vi "UHR-Fleezers Control (host) - 11.9c.vi"() -> ()   [LabVIEW 2014] (continued)
                  }
                  frame True {
                    n2358 = flat-sequence {
                      tunnel: w3436 -> [w3439]
                      tunnel: [w3437] -> w3435
                      tunnel: w3435 -> [w3441]
                      frame #0 {
                        w3438 = TRUE ("Resize to Image Size? (Y)")
                        w3437 = 0 ("Window Number (0...15)")
                        n2359 = call "IMAQ WindNonTearing"("Window Number"=w3437, "NonTearing? (True)"=w3438) -> ()  [unwired: 8 in, 2 out]
                        n2360 = call "IMAQ WindDraw"("Resize to Image Size? (Y)"=w3438, "Window Number (0...15)"=w3437, "Image"=w3439) -> ()  [unwired: 7 in, 2 out]
                      }
                      frame #1 {
                        n2361 = call "IMAQ WindSize"("Scrollbars? (N)"=FALSE, "Width & Height"="Initial Window Size", "Window Number"=w3441) -> ()  [unwired: 3 in, 3 out]
                        n2362 = call "IMAQ WindMove"("Window Number (0...15)"=w3441, "Coordinates (screen)"="Initial Window Position") -> ()  [unwired: 3 in, 2 out]
                      }
                    }
                  }
                }
              }
              frame Enabled {
              }
            }
            n2363 = To Unsigned Byte Integer(number=w3386) -> (unsigned 8bit integer=w3385:u8[][])
            n2364 = call "IMAQ ArrayToImage"("Image Pixels (U8)"=w3385, "Image"=w3382) -> ("Image Out"=w3380:T2)  [unwired: 4 in, 5 out]
            n2365 = case shown="True" "Save Video" {
              tunnel: w3387 -> [_ w3445]
              tunnel: w3380 -> [_ w3444]
              frame False {
              }
              frame True {
                n2366 = call "IMAQ AVI Write Frame"("Image"=w3444, "Avi Refnum"=w3445) -> ()  [unwired: 2 in, 8 out]
              }
            }
            n2367 = case shown="True" "Save Image" {
              tunnel: w3385 -> [_ w3460]
              tunnel: w3384 -> [_ w3459]
              frame False {
              }
              frame True {
                n2368 = call <vilib>:"Flatten Pixmap.vi"("colors"=w3459, "8-bit pixmap"=w3460) -> ("image data"=w3466:T35)  [unwired: 4 in, 5 out]
                n2369 = call "Create new save file.vi"("Insert"="video_frame_" ("string"), "Ext"=".bmp" ("string"), "Index In"="Image Index") -> ("Path Out"=w3462:path, "Index Out"=w3467:dbl)
                n2370 = Increment(x=w3467) -> (x+1=w3461:dbl)
                n2371 = local write "Image Index"(w3461) -> ()
                n2372 = call <vilib>:"Write BMP File.vi"("image data"=w3466, "path to BMP file"=w3462) -> ()  [unwired: 1 in, 9 out]
              }
            }
            n2373 = case shown="True" "Target" {
              tunnel: w3380 -> [w3406 w3410]
              tunnel: [w3406 w3408] -> w3379
              frame False {
              }
              frame True {
                n2374 = local read "Target coordinates"() -> (w3407:cluster{"X1":dbl, "Y1":dbl, "X2":dbl, "Y2":dbl})
                n2375 = call "IMAQ Overlay Oval"("Color"=u32 16711680, "Bounding Rectangle"=w3407, "Image"=w3410) -> ("Image Out"=w3408:T2)  [unwired: 7 in, 1 out]
              }
            }
            "Primary Video Display" <- w3379
          }
        }
        n2376 = node-c288(w3341) -> ()  [unwired: 1 out]
      }
      n2377 = node-c288(w3325) -> ()  [unwired: 1 out]
      n2378 = call "DMR_CloseDevice2.vi"("driver handle IN"=w3330) -> ()  [unwired: 1 in, 4 out]
    }
    frame #4 {
      n2379 = call "DMR_Close.vi"() -> ()  [unwired: 1 out]
    }
  }
  n2380 = local write "Offset (nm)"(0.0 ("Offset (nm)")) -> ()
  n2381 = local write "Bead Mean (nm)"(0.0 ("Bead Mean (nm)")) -> ()
  n2382 = local write "Total Volume\nFlowed P1 (uL)"(w26) -> ()
  n2383 = local write "Total Volume\nFlowed Samp (uL)"(w26) -> ()
  n2384 = local write "Total Volume\nFlowed P3 (uL)"(w26) -> ()
  n2385 = node-c288(i64 1 ("Period"), 1 ("Processor")) -> (w200:T22)  [unwired: 2 out]
  n2386 = timed-loop "Acquire Data" {
    tunnel: w32 -> [w3775]
    tunnel: w79 -> [w3774]
    tunnel: [w3804] -> w293
    tunnel: [w3799] -> w291
    timing: w200 -> [_]
    timing-out: [_] -> w199
    tunnel: w98 -> [w3614]
    stop <- "Stop All" stop-if-true
    w3532 = "Initialize"
    w3601 = "NI_ChannelName" ("name")
    # "I think that the conversion\nfrom 'wiggle amp' to nm\nis 0.277 nm/input. So, 1000\nfor an input is 277 nm."
    n2387 = node-c288() -> ()  [unwired: 2 out]
    n2388 = First Call?() -> (First Call?: T/F=w3567:bool)
    n2389 = Or(x="Reset", y=w3567) -> (x .or. y?=w3568:bool)
    n2390 = local read "Flushing P1"() -> (w3487:bool)
    n2391 = case "Reset data stream" shown="True" w3568 {
      tunnel: w3775 -> [w4844 w4852]
      tunnel: w3774 -> [w4843 w4851]
      tunnel: [w4844 w4846] -> w3480
      tunnel: [w4843 w4845] -> w3770
      frame False {
      }
      frame True {
        w4849 = TRUE ("AI to FIFO")
        n2392 = local write "Overflow (data lost)"(FALSE ("Overflow (data lost)")) -> ()
        n2393 = call "reset FPGA DMA.vi"("error in"=w4851, "FPGA VI Reference In"=w4852) -> ("error out"=w4847:errorcluster, "FPGA VI Reference Out"=w4848:T20)
        n2394 = xnode "Read/Write Control"("FPGA VI Reference In"=w4848, "error in"=w4847, "AI to FIFO"=w4849, "APD to FIFO"=w4849) -> ("FPGA VI Reference Out"=w4846:T20, "error out"=w4845:errorcluster)
      }
    }
    n2395 = case shown="True" w3487 {
      frame False {
      }
      frame True {
        n2396 = local read "Flush rate (uL/m) P1"() -> (w3877:dbl)
        n2397 = local read "HP1 Flush Time (s)"() -> (w3883:dbl)
        n2398 = local read "DMA Update Period (s)"() -> (w3870:dbl)
        n2399 = Divide(x=w3877, y=60.0) -> (x/y=w3869:dbl)
        n2400 = feedback #4(0.0) -> (w3872:dbl)
        n2401 = Divide(x=w3883, y=w3870) -> (x/y=w3875:dbl)
        n2402 = feedback #5(0) -> (w3881:i32)
        n2403 = Increment(x=w3881) -> (x+1=w3874:i32)
        n2404 = Multiply(x=w3870, y=w3869) -> (x*y=w3868:dbl)
        n2405 = Greater?(x=w3874, y=w3875) -> (0:w3880:bool)
        n2406 = Compound Arithmetic op=MULTIPLY(w3870, w3874, w3869) -> (→"P1 Flush Volume (uL)":dbl)
        n2407 = Divide(x=w3874, y=w3875) -> (x/y=→"P1 Flushing Bar":dbl)
        n2408 = Add(x=w3868, y=w3872) -> (x+y=w3871:dbl)
        "Total Volume\nFlowed P1 (uL)" <- w3871
        n2409 = feedback-in #4(w3871) -> ()
        n2410 = case shown="True" w3880 {
          tunnel: w3874 -> [w3884 _]
          tunnel: [w3884 0] -> w3879
          frame False {
          }
          frame True {
            w3885 = FALSE ("Flushing P1")
            n2411 = local write "Inject Pump 1"(w3885) -> ()
            n2412 = local write "Flushing P1"(w3885) -> ()
            n2413 = property on="Clear Volume P1" class="Bool (strict)"("Val(Sgnl)"=TRUE ("Value (Signaling)")) -> ()  [unwired: 2 in, 2 out]
          }
        }
        n2414 = feedback-in #5(w3879) -> ()
      }
    }
    n2415 = Or(x="Start AOD Scan", y="Trap Raster Scan") -> (x .or. y?=w3722:bool)
    n2416 = case "Start AOM raster scan" shown="True" w3722 {
      tunnel: w3480 -> [w4694 w4704]
      tunnel: w3770 -> [w4693 w4703]
      tunnel: [w4694 w4697] -> w3472
      tunnel: [w4693 w4696] -> w3769
      frame False {
      }
      frame True {
        n2417 = case shown="True" "Restart DMA? (AOD)" {
          tunnel: [w4742 w4744] -> w4698
          tunnel: [w4741 w4743] -> w4699
          tunnel: w4704 -> [w4742 w4746]
          tunnel: w4703 -> [w4741 w4745]
          frame False {
          }
          frame True {
            n2418 = local write "Overflow (data lost)"(FALSE ("Overflow (data lost)")) -> ()
            n2419 = call "reset FPGA DMA.vi"("error in"=w4745, "FPGA VI Reference In"=w4746) -> ("error out"=w4743:errorcluster, "FPGA VI Reference Out"=w4744:T20)
          }
        }
        n2420 = local write "Trap Raster Scan"(FALSE ("Trap Raster Scan")) -> ()
        n2421 = case shown="False" "Move MCL Also?" {
          tunnel: w4699 -> [w4708 w4736]
          tunnel: w4698 -> [w4709 w4737]
          tunnel: [w4707 w4740] -> w4697
          tunnel: [w4706 w4739] -> w4696
          frame False {
            w4705 = TRUE ("AI to FIFO")
            n2422 = xnode "Read/Write Control"("FPGA VI Reference In"=w4709, "error in"=w4708, "AI to FIFO"=w4705, "APD to FIFO"=w4705, "Start scan"=w4705) -> ("FPGA VI Reference Out"=w4707:T20, "error out"=w4706:errorcluster)
          }
          frame True {
            w4733 = FALSE ("1D or 2D Scan?")
            w4738 = TRUE ("AI to FIFO")
            # "Count for MCL loop"
            # "N total cycles"
            # "N steps"
            # "V_int"
            n2423 = local read "Scan Range (nm)"() -> (w4715:dbl)
            n2424 = local read "Number of F/B Scans (AOD)"() -> (w4732:u16)
            n2425 = Sign(1:w4715) -> (0:w4714:dbl)
            n2426 = Compound Arithmetic op=MULTIPLY(w4715, "MCL Step Position Ratio", "MCL/AOM Scale Tweak") -> (w4719:dbl)
            n2427 = Negate(x=w4714) -> (-x=w4711:dbl)
            n2428 = Multiply(x=w4711, y="MCL Step Increment (V_int)") -> (x*y=w4713:dbl)
            n2429 = Divide(x=w4719, y="MCL X Cal (nm/V)") -> (x/y=w4725:dbl)
            n2430 = Multiply(x=32767.0 ("y"), y=w4725) -> (x*y=w4731:dbl)
            n2431 = local read "Total Counts (ticks)"() -> (w4716:u32)
            n2432 = local read "Cycles/step (AOD)"() -> (w4727:u64)
            n2433 = local read "Scan steps (AOD)"() -> (w4728:u64)
            n2434 = Divide(x=w4731, y=10.0) -> (x/y=w4724:dbl)
            n2435 = Divide(x=w4724, y="MCL Step Increment (V_int)") -> (x/y=w4722:dbl)
            n2436 = Absolute Value(x=w4722) -> (abs(x)=w4710:dbl)
            n2437 = Compound Arithmetic op=MULTIPLY(w4728, w4727, w4716) -> (w4723:u64)
            n2438 = local write "wait to reset values"(w4738) -> ()
            n2439 = local write "MCL Scanning"(w4738) -> ()
            n2440 = Divide(x=w4723, y=w4710) -> (x/y=w4720:dbl)
            "MCL Count" <- w4720
            n2441 = xnode "Read/Write Control"("FPGA VI Reference In"=w4737, "error in"=w4736, "Scan steps (MCL)"=w4710, "Number of scans (MCL)"=w4732, "Cycles per step (MCL)"=u64 1, "Scan freq.  increment (MCL)"=w4713, "1D or 2D Scan?"=w4733, "MCL Scan Axis"=w4733, "Cont. Scan (MCL)"=w4733, "MCL count"=w4720) -> ("FPGA VI Reference Out"=w4735:T20, "error out"=w4734:errorcluster)
            n2442 = xnode "Read/Write Control"("FPGA VI Reference In"=w4735, "error in"=w4734, "AI to FIFO"=w4738, "APD to FIFO"=w4738, "Start scan"=w4738, "Start scan (MCL)"=w4738) -> ("FPGA VI Reference Out"=w4740:T20, "error out"=w4739:errorcluster)
          }
        }
        "Raster Scanning..." <- TRUE ("Scanning...")
      }
    }
    n2443 = local read "Flushing P3"() -> (w3488:bool)
    n2444 = case "Keep track of when Harvard Pump 3 is done flushing" shown="True" w3488 {
      frame False {
      }
      frame True {
        n2445 = local read "Flush rate (uL/m) P3"() -> (w3896:dbl)
        n2446 = local read "DMA Update Period (s)"() -> (w3890:dbl)
        n2447 = local read "HP3 Flush Time (s)"() -> (w3904:dbl)
        n2448 = Divide(x=w3896, y=60.0) -> (x/y=w3891:dbl)
        n2449 = feedback #6(0) -> (w3902:i32)
        n2450 = Increment(x=w3902) -> (x+1=w3897:i32)
        n2451 = Divide(x=w3904, y=w3890) -> (x/y=w3898:dbl)
        n2452 = Multiply(x=w3890, y=w3891) -> (x*y=w3889:dbl)
        n2453 = Greater?(x=w3897, y=w3898) -> (0:w3901:bool)
        n2454 = feedback #7(0.0) -> (w3892:dbl)
        n2455 = Compound Arithmetic op=MULTIPLY(w3890, w3897, w3891) -> (→"P3 Flush Volume (uL)":dbl)
        n2456 = case shown="True" w3901 {
          tunnel: w3897 -> [w3905 _]
          tunnel: [w3905 0] -> w3900
          frame False {
          }
          frame True {
            w3906 = FALSE ("Flushing P3")
            n2457 = local write "Inject Pump 3"(w3906) -> ()
            n2458 = local write "Flushing P3"(w3906) -> ()
            n2459 = property on="Clear Volume P3" class="Bool (strict)"("Val(Sgnl)"=TRUE ("Value (Signaling)")) -> ()  [unwired: 2 in, 2 out]
          }
        }
        n2460 = feedback-in #6(w3900) -> ()
        n2461 = Divide(x=w3897, y=w3898) -> (x/y=→"P3 Flushing Bar":dbl)
        n2462 = Add(x=w3889, y=w3892) -> (x+y=w3893:dbl)
        "Total Volume\nFlowed P3 (uL)" <- w3893
        n2463 = feedback-in #7(w3893) -> ()
      }
    }
    n2464 = And(x="Save scans", y=w3722) -> (x .and. y?=w3768:bool)
    n2465 = local read "Flushing samp"() -> (w3481:bool)
    n2466 = case shown="True" w3481 {
      frame False {
      }
      frame True {
        n2467 = local read "DMA Update Period (s)"() -> (w3849:dbl)
        n2468 = local read "Flush rate (mL/m)"() -> (w3861:dbl)
        n2469 = local read "Samp Flush Time (s)"() -> (w3862:dbl)
        n2470 = Divide(x=w3861, y=60.0) -> (x/y=w3848:dbl)
        n2471 = feedback #8(0) -> (w3854:i32)
        n2472 = Increment(x=w3854) -> (x+1=w3853:i32)
        n2473 = Divide(x=w3862, y=w3849) -> (x/y=w3858:dbl)
        n2474 = Multiply(x=w3849, y=w3848) -> (x*y=w3847:dbl)
        n2475 = Greater?(x=w3853, y=w3858) -> (0:w3857:bool)
        n2476 = feedback #9(0.0) -> (w3850:dbl)
        n2477 = Compound Arithmetic op=MULTIPLY(w3849, w3853, w3848) -> (→"Samp Volume (uL)":dbl)
        n2478 = Divide(x=w3853, y=w3858) -> (x/y=→"Samp flush bar":dbl)
        n2479 = case shown="True" w3857 {
          tunnel: [w3863 0] -> w3856
          tunnel: w3853 -> [w3863 _]
          frame False {
          }
          frame True {
            w3866 = FALSE ("Flushing samp")
            n2480 = local write "Sample Channel\nFlow"(w3866) -> ()
            n2481 = local write "Flushing samp"(w3866) -> ()
            n2482 = property on="Clear Volume" class="Bool (strict)"("Val(Sgnl)"=TRUE) -> ()  [unwired: 2 in, 2 out]
          }
        }
        n2483 = feedback-in #8(w3856) -> ()
        n2484 = Add(x=w3847, y=w3850) -> (x+y=w3851:dbl)
        "Total Volume\nFlowed Samp (uL)" <- w3851
        n2485 = feedback-in #9(w3851) -> ()
      }
    }
    n2486 = Compound Arithmetic op=OR("Start MCL Scan", "Confocal\nImage", "Confocal\nLinescan") -> (w3720:bool)
    n2487 = And(x="Save Data (MCL)", y=w3720) -> (x .and. y?=w3767:bool)
    n2488 = case "Start MCL raster scan" shown="True" w3720 {
      tunnel: w3472 -> [w4311 w4327]
      tunnel: w3769 -> [w4310 w4326]
      tunnel: [w4311 w4322] -> w3479
      tunnel: [w4310 w4321] -> w3477
      tunnel: [FALSE w4320] -> w3753
      tunnel: "Start MCL Scan" -> [_ w4315]
      tunnel: "Confocal\nImage" -> [_ w4314]
      tunnel: "Confocal\nLinescan" -> [_ _]
      frame False {
      }
      frame True {
        w4320 = TRUE
        n2489 = case shown="True" "Restart DMA? (MCL)" {
          tunnel: [w4372 w4374] -> w4325
          tunnel: [w4371 w4373] -> w4324
          tunnel: w4327 -> [w4372 w4377]
          tunnel: w4326 -> [w4371 w4376]
          frame False {
          }
          frame True {
            n2490 = call "reset FPGA DMA.vi"("error in"=w4376, "FPGA VI Reference In"=w4377) -> ("error out"=w4373:errorcluster, "FPGA VI Reference Out"=w4374:T20)
            n2491 = local write "Overflow (data lost)"(FALSE ("Overflow (data lost)")) -> ()
          }
        }
        n2492 = case shown="False" w4315 {
          selector: w4315 -> [_ w4331]
          tunnel: w4314 -> [w4330 _]
          tunnel: [w4330 w4331] -> w4313
          frame False {
            n2493 = property on="2D or 1D Scan" class="Bool (strict)"("Val(Sgnl)"=w4330) -> ()  [unwired: 2 in, 2 out]
            n2494 = property on="Confocal\nImage" class="Bool (strict)"("Value"=FALSE ("Start Confocal Map")) -> ()  [unwired: 2 in, 2 out]
          }
          frame True {
          }
        }
        n2495 = local write "MCL Scanning"(w4320) -> ()
        n2496 = local read "AO1"() -> (w4317:dbl)
        n2497 = local read "AO2"() -> (w4316:dbl)
        n2498 = case shown="True" "Center Scan" {
          tunnel: w4325 -> [w4338 w4370]
          tunnel: w4324 -> [w4337 w4369]
          tunnel: [w4336 w4368] -> w4322
          tunnel: [w4335 w4367] -> w4321
          tunnel: [w4333 w4354] -> w4319
          tunnel: [w4332 w4353] -> w4318
          tunnel: w4317 -> [w4333 w4359]
          tunnel: w4316 -> [w4332 w4362]
          tunnel: w4313 -> [_ _]
          frame False {
            w4334 = TRUE ("AI to FIFO")
            n2499 = xnode "Read/Write Control"("FPGA VI Reference In"=w4338, "error in"=w4337, "AI to FIFO"=w4334, "APD to FIFO"=w4334, "Start scan (MCL)"=w4334) -> ("FPGA VI Reference Out"=w4336:T20, "error out"=w4335:errorcluster)
          }
          frame True {
            w4366 = TRUE ("AI to FIFO")
            n2500 = local read "Scan steps (MCL)"() -> (w4345:u64)
            n2501 = local read "Scan lines (y)"() -> (w4341:u64)
            n2502 = local read "Fast Scan Dir"() -> (w4352:bool)
            n2503 = local read "Actual MCL Inc (V)"() -> (w4342:dbl)
            n2504 = Decrement(x=w4341) -> (x-1=w4340:u64)
            n2505 = Decrement(x=w4345) -> (x-1=w4344:u64)
            n2506 = Multiply(x=w4342, y=w4340) -> (x*y=w4339:dbl)
            n2507 = Divide(x=w4339, y=2.0) -> (x/y=w4349:dbl)
            n2508 = Multiply(x=w4342, y=w4344) -> (x*y=w4343:dbl)
            n2509 = Divide(x=w4343, y=2.0) -> (x/y=w4348:dbl)
            n2510 = Select(t=w4348, s=w4352, f=w4349) -> (s? t:f=w4347:dbl)
            n2511 = Select(t=w4349, s=w4352, f=w4348) -> (s? t:f=w4351:dbl)
            n2512 = Subtract(x=w4359, y=w4351) -> (x-y=w4350:dbl)
            n2513 = Subtract(x=w4362, y=w4347) -> (x-y=w4346:dbl)
            n2514 = local read "2D or 1D Scan"() -> (w4364:bool)
            n2515 = Not(x=w4352) -> (.not. x?=w4358:bool)
            n2516 = Not(x=w4364) -> (.not. x?=w4360:bool)
            n2517 = And(x=w4352, y=w4360) -> (x .and. y?=w4361:bool)
            n2518 = And(x=w4360, y=w4358) -> (x .and. y?=w4363:bool)
            n2519 = Select(t=w4362, s=w4363, f=w4346) -> (s? t:f=w4353:dbl)
            n2520 = Select(t=w4359, s=w4361, f=w4350) -> (s? t:f=w4354:dbl)
            n2521 = call "Volt to I16.vi"("Voltage In"=w4354) -> ("I16 Voltage Out"=w4357:i16)
            n2522 = call "Volt to I16.vi"("Voltage In"=w4353) -> ("I16 Voltage Out"=w4356:i16)
            n2523 = xnode "Read/Write Control"("FPGA VI Reference In"=w4370, "error in"=w4369, "AI to FIFO"=w4366, "APD to FIFO"=w4366, "Start scan (MCL)"=w4366, "AO1"=w4357, "AO2"=w4356) -> ("FPGA VI Reference Out"=w4368:T20, "error out"=w4367:errorcluster)
          }
        }
        "Initial Y" <- w4319
        "Initial X" <- w4318
        n2524 = local write "Tab Control 6"(T3."Imaging" ("Tab Control 6")) -> ()
        "wait to reset values" <- w4320
      }
    }
    n2525 = case shown="True" "Wiggle" {
      selector: "Wiggle" -> [w3820 _]
      tunnel: w3479 -> [w3822 w3835]
      tunnel: [w3819 w3838] -> w3478
      tunnel: w3477 -> [w3821 w3833]
      tunnel: [w3818 w3837] -> w3476
      frame False {
        n2526 = xnode "Read/Write Control"("FPGA VI Reference In"=w3822, "error in"=w3821, "Wiggle trap 1"=w3820) -> ("FPGA VI Reference Out"=w3819:T20, "error out"=w3818:errorcluster)
      }
      frame True {
        w3827 = FALSE ("Abort wiggle")
        w3831 = TRUE
        n2527 = local read "Restart DMA? (AOD)"() -> (w3836:bool)
        n2528 = case shown="True" w3836 {
          tunnel: w3835 -> [w3840 w3845]
          tunnel: [w3840 w3844] -> w3834
          tunnel: w3833 -> [w3839 w3843]
          tunnel: [w3839 w3842] -> w3832
          frame False {
          }
          frame True {
            n2529 = local write "Overflow (data lost)"(FALSE) -> ()
            n2530 = call "reset FPGA DMA.vi"("error in"=w3843, "FPGA VI Reference In"=w3845) -> ("error out"=w3842:errorcluster, "FPGA VI Reference Out"=w3844:T20)
          }
        }
        n2531 = local write "Wiggle"(FALSE) -> ()
        n2532 = xnode "Read/Write Control"("FPGA VI Reference In"=w3834, "error in"=w3832, "AI to FIFO"=w3831, "APD to FIFO"=w3831, "Wiggle trap 1"="Wiggle T1", "Wiggle freq 1 (Hz)"="Wiggle freq 1 (Hz)", "Wiggle amp 1"="Wiggle amp 1 (units?)", "Abort wiggle 1"=w3827, "Wiggle trap 2"="Wiggle T2", "Abort wiggle 2"=w3827, "Wiggle freq 2 (Hz)"="Wig Freq 2 (Hz)", "Wiggle amp 2"="Wig amp 2") -> ("FPGA VI Reference Out"=w3838:T20, "error out"=w3837:errorcluster)
      }
    }
    n2533 = local read "Trap Pos Elements/DMA read"() -> (w3610:u32)
    n2534 = local read "Trap AI Elements/DMA read"() -> (w3683:u32)
    n2535 = local read "APD Elements/DMA read"() -> (w3649:u32)
    n2536 = xnode "Get APD Data"("FPGA VI Reference In"=w3478, "error in"=w3476, "Number of Elements"=w3649, "Timeout (ms)"=-1) -> ("Data"=w3648:u32[], "Elements Remaining"=→"APD FIFO Elements Remaining":u32)  [unwired: 2 out]
    n2537 = xnode "Invoke Method"("FPGA VI Reference In"=w3478, "error in"=w3476, "Number of Elements"=w3610, "Timeout (ms)"=-1) -> ("Data"=w3574:u16[], "Elements Remaining"=→"Trap Pos FIFO El Remaining":u32)  [unwired: 2 out]
    n2538 = xnode "Get Trap Data"("FPGA VI Reference In"=w3478, "error in"=w3476, "Number of Elements"=w3683, "Timeout (ms)"=-1 ("Timeout")) -> ("FPGA VI Reference Out"=w3509:T20, "error out"=w3508:errorcluster, "Data"=w3575:i16[], "Elements Remaining"=w3812:u32)
    "FIFO El. Rem." <- w3812
    n2539 = local read "Trap AI FIFO Depth"() -> (w3814:u32)
    n2540 = Subtract(x=w3814, y=w3683) -> (x-y=w3813:u32)
    n2541 = Decimate 1D Array(w3574) -> (w3571:u16[], w3573:u16[], w3572:u16[])
    n2542 = Divide(x=w3812, y=w3813) -> (x/y=w3811:dbl)
    "Buffer Status" <- w3811
    n2543 = To Unsigned Long Integer(number=w3571) -> (unsigned 32bit integer=w3570:u32[])
    n2544 = Join Numbers(hi=w3573, lo=w3572) -> ((hi.lo)=w3569:u32[])
    n2545 = Equal?(x=w3811, y=1.0) -> (x = y?=w3809:bool)
    n2546 = Join Numbers(hi=w3570, lo=w3569) -> ((hi.lo)=w3563:u64[])
    n2547 = call "IR AOM word to freq - vec.vi"("Frequency Word In (double vec)"=w3563) -> ("Frequency Out"=w3609:dbl[])
    n2548 = case "Alert buffer overflow" shown="True" w3809 {
      frame False {
      }
      frame True {
        n2549 = call <vilib>:"Beep.vi"() -> ()  [unwired: 3 in, 9 out]
        "Overflow (data lost)" <- TRUE ("Overflow (data lost)")
      }
    }
    n2550 = Decimate 1D Array(w3609) -> (w3608:dbl[], w3607:dbl[])
    n2551 = Build Array(w3608, w3607) -> (w3606:dbl[][])
    n2552 = local read "Trap Sets"() -> (w3682:u32)
    n2553 = case "Deinterlace trap data, average down PSD" shown="2" w3682 {
      tunnel: w3575 -> [w4407 w4472]
      tunnel: [w4404 w4469] -> w3675
      tunnel: [w4407 w4471] -> w3566
      tunnel: "Detector Type" -> [w4406 w4467]
      tunnel: [w4405 w4470] -> w3674
      tunnel: [w4403 w4468] -> w3786
      frame 1, Default {
        n2554 = Divide(x=w4407, y=3276.7) -> (x/y=w4408:dbl[])
        n2555 = Decimate 1D Array(w4408) -> (w4417:dbl[], w4416:dbl[], w4415:dbl[], w4414:dbl[], w4413:dbl[], w4412:dbl[], w4411:dbl[], w4410:dbl[])
        n2556 = case shown="\"IR-QPD + PSD + FB-QPD position\"" w4406 {
          tunnel: w4417 -> [w4441 w4466]
          tunnel: w4416 -> [w4440 w4465]
          tunnel: w4415 -> [w4425 w4443]
          tunnel: w4414 -> [w4426 w4453]
          tunnel: w4413 -> [w4439 w4464]
          tunnel: w4412 -> [w4438 w4463]
          tunnel: w4411 -> [w4422 w4444]
          tunnel: w4410 -> [w4421 w4442]
          tunnel: [w4420 w4450] -> w4405
          tunnel: [w4419 w4449] -> w4404
          tunnel: [w4418 w4448] -> w4403
          frame "IR-QPD + PSD + FB-QPD", Default {
            w4418 = 0  # Channel pattern
            n2557 = Divide(x=w4441, y=w4426) -> (x/y=w4428:dbl[])
            n2558 = Divide(x=w4440, y=w4426) -> (x/y=w4427:dbl[])
            n2559 = Divide(x=w4439, y=w4422) -> (x/y=w4424:dbl[])
            n2560 = Divide(x=w4438, y=w4421) -> (x/y=w4423:dbl[])
            n2561 = Build Array(w4428, w4427, w4426, w4425, w4424, w4423, w4422, w4421) -> (w4419:dbl[][])
            n2562 = Bundle("T1 Y", "T1 X", "T1 Sum", "FB Sum", "PSD Y", "PSD X", "PSD Y Sum", "PSD X Sum") -> (w4437:T42)  [unwired: 1 out]
            n2563 = Cluster To Array(cluster=w4437) -> (array=w4420:string[])
          }
          frame "IR-QPD + PSD + FB-QPD position" {
            w4448 = 3  # Channel pattern
            n2564 = Negate(x=w4444) -> (-x=w4445:dbl[])
            n2565 = Divide(x=w4466, y=w4453) -> (x/y=w4455:dbl[])
            n2566 = Divide(x=w4465, y=w4453) -> (x/y=w4454:dbl[])
            n2567 = Divide(x=w4464, y=w4444) -> (x/y=w4452:dbl[])
            n2568 = Divide(x=w4463, y=w4445) -> (x/y=w4451:dbl[])
            n2569 = Build Array(w4455, w4454, w4453, w4442, w4443, w4452, w4451, w4444) -> (w4449:dbl[][])
            n2570 = Bundle("T1 Y", "T1 X", "T1 Sum", "FB X", "FB Sum", "PSD Y", "PSD X", "PSD Y Sum") -> (w4462:T42)  [unwired: 1 out]
            n2571 = Cluster To Array(cluster=w4462) -> (array=w4450:string[])
          }
        }
      }
      frame 2 {
        n2572 = case shown="\"IR-QPD + PSD + FB-QPD\", Default" w4467 {
          tunnel: w4472 -> [w4534 w4601 w4672]
          tunnel: [w4473 w4592 w4603] -> w4471
          tunnel: [w4500 w4583 w4650] -> w4470
          tunnel: [w4499 w4546 w4617] -> w4469
          tunnel: [w4493 w4581 w4648] -> w4468
          frame "IR-QPD + PSD + FB-QPD", Default {
            w4493 = 1  # Channel pattern
            # "time average x2 the 4th signal and the 4 psd signals (detection laser)"
            # "deinterlace 3 signals from qpd"
            n2573 = Decimate 1D Array(w4534) -> (w4533:i16[], w4532:i16[], w4498:i16[], w4531:i16[], w4521:i16[], w4519:i16[], w4518:i16[], w4516:i16[])
            n2574 = Decimate 1D Array(w4498) -> (w4497:i16[], w4496:i16[])
            n2575 = Decimate 1D Array(w4533) -> (w4530:i16[], w4502:i16[])
            n2576 = Decimate 1D Array(w4532) -> (w4529:i16[], w4527:i16[])
            n2577 = Decimate 1D Array(w4531) -> (w4528:i16[], w4526:i16[])
            n2578 = call "downsample 1D array - double.vi"("Ave N"=2.0, "Array In"=w4521) -> ("Array Out"=w4520:dbl[])  [unwired: 1 out]
            n2579 = call "downsample 1D array - double.vi"("Ave N"=2.0, "Array In"=w4519) -> ("Array Out"=w4501:dbl[])  [unwired: 1 out]
            n2580 = call "downsample 1D array - double.vi"("Ave N"=2.0, "Array In"=w4518) -> ("Array Out"=w4517:dbl[])  [unwired: 1 out]
            n2581 = call "downsample 1D array - double.vi"("Ave N"=2.0, "Array In"=w4516) -> ("Array Out"=w4515:dbl[])  [unwired: 1 out]
            n2582 = Interleave 1D Arrays(w4530, w4529, w4528, w4502, w4527, w4526, w4497, w4496, w4520, w4501, w4517, w4515) -> (w4514:dbl[])
            n2583 = Divide(x=w4514, y=3276.7) -> (x/y=w4513:dbl[])
            n2584 = Decimate 1D Array(w4513) -> (w4512:dbl[], w4511:dbl[], w4510:dbl[], w4509:dbl[], w4508:dbl[], w4507:dbl[], w4495:dbl[], w4494:dbl[], w4506:dbl[], w4505:dbl[], w4504:dbl[], w4503:dbl[])
            n2585 = Divide(x=w4512, y=w4510) -> (x/y=w4480:dbl[])
            n2586 = Divide(x=w4511, y=w4510) -> (x/y=w4479:dbl[])
            n2587 = Divide(x=w4509, y=w4507) -> (x/y=w4478:dbl[])
            n2588 = Divide(x=w4508, y=w4507) -> (x/y=w4477:dbl[])
            n2589 = Divide(x=w4506, y=w4504) -> (x/y=w4476:dbl[])
            n2590 = Divide(x=w4505, y=w4503) -> (x/y=w4475:dbl[])
            n2591 = Build Array(w4480, w4479, w4510, w4478, w4477, w4507, w4495, w4494, w4476, w4475, w4504, w4503) -> (w4499:dbl[][])
            n2592 = Bundle("T1 Y", "T1 X", "T1 Sum", "T2 Y", "T2 X", "T2 Sum", "T1 FB Sum", "T2 FB Sum", "PSD Y", "PSD X", "PSD Y Sum", "PSD X Sum") -> (w4481:T43)  [unwired: 1 out]
            n2593 = To Word Integer(number=w4514) -> (16bit integer=w4473:i16[])
            n2594 = Cluster To Array(cluster=w4481) -> (array=w4500:string[])
          }
          frame "IR-QPD + PSD + FB-QPD X position" {
            w4581 = 2  # Channel pattern
            # "time average x2 the 3 psd signals (detection laser)"
            # "deinterlace 3 signals from qpds"
            n2595 = Decimate 1D Array(w4601) -> (w4600:i16[], w4599:i16[], w4582:i16[], w4598:i16[], w4544:i16[], w4541:i16[], w4538:i16[], w4569:i16[])
            n2596 = Decimate 1D Array(w4582) -> (w4567:i16[], w4565:i16[])
            n2597 = Decimate 1D Array(w4600) -> (w4597:i16[], w4584:i16[])
            n2598 = Decimate 1D Array(w4599) -> (w4596:i16[], w4594:i16[])
            n2599 = Decimate 1D Array(w4598) -> (w4595:i16[], w4593:i16[])
            n2600 = Decimate 1D Array(w4569) -> (w4568:i16[], w4566:i16[])
            n2601 = call "downsample 1D array - I16.vi"("Ave N"=2.0, "Array In"=w4544) -> ("Array Out"=w4542:i16[])  [unwired: 1 in]
            n2602 = call "downsample 1D array - I16.vi"("Ave N"=2.0, "Array In"=w4538) -> ("Array Out"=w4536:i16[])  [unwired: 1 in]
            n2603 = call "downsample 1D array - I16.vi"("Ave N"=2.0, "Array In"=w4541) -> ("Array Out"=w4539:i16[])  [unwired: 1 in]
            n2604 = Interleave 1D Arrays(w4597, w4596, w4595, w4584, w4594, w4593, w4568, w4567, w4566, w4565, w4542, w4539, w4536) -> (w4592:i16[])
            n2605 = Divide(x=w4592, y=3276.7) -> (x/y=w4591:dbl[])
            n2606 = Decimate 1D Array(w4591) -> (w4590:dbl[], w4589:dbl[], w4588:dbl[], w4587:dbl[], w4586:dbl[], w4585:dbl[], w4557:dbl[], w4555:dbl[], w4554:dbl[], w4552:dbl[], w4551:dbl[], w4550:dbl[], w4547:dbl[])
            n2607 = Negate(x=w4547) -> (-x=w4545:dbl[])
            n2608 = Divide(x=w4551, y=w4547) -> (x/y=w4549:dbl[])
            n2609 = Divide(x=w4550, y=w4545) -> (x/y=w4548:dbl[])
            n2610 = Divide(x=w4590, y=w4588) -> (x/y=w4573:dbl[])
            n2611 = Divide(x=w4589, y=w4588) -> (x/y=w4572:dbl[])
            n2612 = Divide(x=w4587, y=w4585) -> (x/y=w4571:dbl[])
            n2613 = Divide(x=w4586, y=w4585) -> (x/y=w4570:dbl[])
            n2614 = Divide(x=w4557, y=w4555) -> (x/y=w4556:dbl[])
            n2615 = Divide(x=w4554, y=w4552) -> (x/y=w4553:dbl[])
            n2616 = Build Array(w4573, w4572, w4588, w4571, w4570, w4585, w4556, w4555, w4553, w4552, w4549, w4548, w4547) -> (w4546:dbl[][])
            n2617 = Bundle("T1 Y", "T1 X", "T1 Sum", "T2 Y", "T2 X", "T2 Sum", "T1 FB X", "T1 FB Sum", "T2 FB X", "T2 FB Sum", "PSD Y", "PSD X", "PSD Y Sum") -> (w4574:T44)  [unwired: 1 out]
            n2618 = Cluster To Array(cluster=w4574) -> (array=w4583:string[])
          }
          frame "IR-QPD + PSD + FB-QPD XY positions" {
            w4648 = 4  # Channel pattern
            # "time average x2 the 3 psd signals (detection laser)"
            # "deinterlace 3 signals from qpds"
            n2619 = Decimate 1D Array(w4672) -> (w4671:i16[], w4670:i16[], w4649:i16[], w4669:i16[], w4615:i16[], w4661:i16[], w4660:i16[], w4637:i16[])
            n2620 = Decimate 1D Array "Feedback Sum"(w4649) -> (w4633:i16[], w4631:i16[])
            n2621 = Decimate 1D Array "QPD Y"(w4671) -> (w4668:i16[], w4651:i16[])
            n2622 = Decimate 1D Array "QPD X"(w4670) -> (w4667:i16[], w4665:i16[])
            n2623 = Decimate 1D Array "Feedback Y"(w4615) -> (w4614:i16[], w4613:i16[])
            n2624 = Decimate 1D Array "QPD Sum"(w4669) -> (w4666:i16[], w4664:i16[])
            n2625 = Decimate 1D Array "Feedback X"(w4637) -> (w4634:i16[], w4632:i16[])
            n2626 = call "downsample 1D array - double.vi"("Ave N"=2.0, "Array In"=w4661) -> ("Array Out"=w4636:dbl[])  [unwired: 1 out]
            n2627 = call "downsample 1D array - double.vi"("Ave N"=2.0, "Array In"=w4660) -> ("Array Out"=w4635:dbl[])  [unwired: 1 out]
            n2628 = Interleave 1D Arrays(w4668, w4667, w4666, w4651, w4665, w4664, w4614, w4634, w4633, w4613, w4632, w4631, w4636, w4635) -> (w4659:dbl[])
            n2629 = Divide(x=w4659, y=3276.7) -> (x/y=w4658:dbl[])
            n2630 = Decimate 1D Array(w4658) -> (w4657:dbl[], w4656:dbl[], w4655:dbl[], w4654:dbl[], w4653:dbl[], w4652:dbl[], w4610:dbl[], w4624:dbl[], w4608:dbl[], w4609:dbl[], w4622:dbl[], w4606:dbl[], w4620:dbl[], w4618:dbl[])
            n2631 = Negate(x=w4618) -> (-x=w4616:dbl[])
            n2632 = Divide(x=w4620, y=w4616) -> (x/y=w4619:dbl[])
            n2633 = Divide(x=w4609, y=w4606) -> (x/y=w4605:dbl[])
            n2634 = Divide(x=w4610, y=w4608) -> (x/y=w4607:dbl[])
            n2635 = Divide(x=w4657, y=w4655) -> (x/y=w4641:dbl[])
            n2636 = Divide(x=w4656, y=w4655) -> (x/y=w4640:dbl[])
            n2637 = Divide(x=w4654, y=w4652) -> (x/y=w4639:dbl[])
            n2638 = Divide(x=w4653, y=w4652) -> (x/y=w4638:dbl[])
            n2639 = Divide(x=w4624, y=w4608) -> (x/y=w4623:dbl[])
            n2640 = Divide(x=w4622, y=w4606) -> (x/y=w4621:dbl[])
            n2641 = Build Array(w4641, w4640, w4655, w4639, w4638, w4652, w4607, w4623, w4608, w4605, w4621, w4606, w4619, w4618) -> (w4617:dbl[][])
            n2642 = Bundle("T1 Y", "T1 X", "T1 Sum", "T2 Y", "T2 X", "T2 Sum", "T1 FB Y", "T1 FB X", "T1 FB Sum", "T2 FB Y", "T2 FB X", "T2 FB Sum", "PSD X", "PSD Y Sum") -> (w4604:T45)  [unwired: 1 out]
            n2643 = To Word Integer(number=w4659) -> (16bit integer=w4603:i16[])
            n2644 = Cluster To Array(cluster=w4604) -> (array=w4650:string[])
          }
        }
      }
    }
    "AI labels" <- w3674
    n2645 = Decimate 1D Array(w3648) -> (w3672:u32[], w3616:u32[])
    n2646 = local read "DMA Update Period (s)"() -> (w3684:dbl)
    n2647 = Build Array(w3672, w3616) -> (w3750:u32[][])
    n2648 = local read "Data Period (s)"() -> (w3525:dbl)
    n2649 = local read "BD 1 Frequency 2 (MHz)"() -> (w3558:dbl)
    n2650 = local read "BD 1 Frequency 1 (MHz)"() -> (w3559:dbl)
    n2651 = Decimate 1D Array(w3566) -> (w3589:i16[], w3588:i16[], w3586:i16[], w3585:i16[])  [unwired: 9 out]
    n2652 = To Double Precision Float(number=w3750) -> (double precision float=w3751:dbl[][])
    n2653 = local read "APD Integration Time (s)"() -> (w3629:dbl)
    n2654 = Multiply(x=w3525, y="Trap Pos. Disp. Downsample") -> (x*y=w3523:dbl)
    n2655 = Divide(x=w3589, y=w3588) -> (x/y=w3590:dbl[])
    n2656 = Divide(x=w3586, y=w3585) -> (x/y=w3587:dbl[])
    n2657 = feedback #10(0.0) -> (w3603:dbl)
    n2658 = Add(x=w3684, y=w3603) -> (x+y=w3788:dbl)
    n2659 = feedback-in #10(w3788) -> ()
    n2660 = local read "AOM X Cal (nm/MHz)"() -> (w3556:dbl)
    n2661 = To Time Stamp(1:w3603) -> (0:w3602:timestamp)
    n2662 = Split 1D Array(array=w3590, index="N El. to Ave.") -> (second subarray=w3593:dbl[])  [unwired: 1 out]
    n2663 = Split 1D Array(array=w3587, index="N El. to Ave.") -> (second subarray=w3592:dbl[])  [unwired: 1 out]
    n2664 = Multiply(x=w3525, y="Trap Disp. Downsample") -> (x*y=w3604:dbl)
    "Display Period (s)" <- w3604
    n2665 = for "Trap AI" {
      tunnel: [w4402] -> w3782 mode=indexing
      tunnel: w3602 -> [w4392]
      tunnel: "Trap Disp. Downsample" -> [w4400]
      tunnel: w3675 -> [w4398] mode=indexing
      tunnel: w3525 -> [w4397]
      tunnel: w3674 -> [w4396] mode=indexing
      tunnel: w3601 -> [w4395]
      tunnel: [w4394] -> w3640 mode=indexing
      tunnel: w3604 -> [w4393]
      workers-P: _ -> [_]
      n2666 = Bundle By Name("Y"=w4398, "dt"=w4397) -> (w4399:waveform(dbl))  [unwired: 1 out]
      n2667 = Set Waveform Attribute(5:w4396, 6:w4395, 7:w4399) -> (3:w4394:waveform(dbl))  [unwired: 1 in, 2 out]
      n2668 = call "downsample 1D array - double.vi"("Ave N"=w4400, "Array In"=w4398) -> ("Array Out"=w4401:dbl[])  [unwired: 1 out]
      n2669 = Bundle By Name(cluster=w4394, "t0"=w4392, "Y"=w4401, "dt"=w4393) -> (w4402:waveform(dbl))
    }
    n2670 = Bundle("BD 1 Frequency 1 (MHz)"=w3559, "BD 1 Frequency 2 (MHz)"=w3558) -> (w3560:T46)  [unwired: 1 out]
    n2671 = call-poly <vilib>:"Mean.vi"("X"=w3592) -> ("mean"=w3580:dbl)  [unwired: 1 out]
    n2672 = call-poly <vilib>:"Mean.vi"("X"=w3593) -> ("mean"=w3581:dbl)  [unwired: 1 out]
    n2673 = Reciprocal(x=w3604) -> (1/x=→"Trap Disp. Freq. (Hz)":dbl)
    n2674 = Cluster To Array(cluster=w3560) -> (array=w3557:dbl[])
    n2675 = local read "Trap X AI1 (DMA)"() -> (w3591:T13)
    n2676 = local read "Data points/scans (MCL)"() -> (w3762:dbl)
    n2677 = To Fixed-Point(number=w3580) -> (fixed-point=w3578:fxp<+/-,16,1>)  [unwired: 1 in]
    n2678 = To Fixed-Point(number=w3581) -> (fixed-point=w3579:fxp<+/-,16,1>)  [unwired: 1 in]
    n2679 = Bundle("Trap 1 Pos.", "Trap 2 Pos.") -> (w3600:cluster{string, string})  [unwired: 1 out]
    n2680 = Bundle By Name(cluster=w3591, "Set 1"=w3579, "Set 2"=w3578) -> (→"Trap X AI1 (DMA)":T13)
    n2681 = Cluster To Array(cluster=w3600) -> (array=w3597:string[])
    n2682 = Bundle("APD 1", "APD 2") -> (w3781:cluster{string, string})  [unwired: 1 out]
    n2683 = Select(t=-1.0, s="Negate Y Axis", f=1.0) -> (s? t:f=w3542:dbl)
    n2684 = for "Trap Position" {
      tunnel: w3606 -> [w4034] mode=indexing
      tunnel: "Trap Pos. Disp. Downsample" -> [w4033]
      tunnel: w3523 -> [w4031]
      tunnel: w3602 -> [w4030]
      tunnel: w3601 -> [w4028]
      tunnel: w3597 -> [w4027] mode=indexing
      tunnel: [w4026] -> w3512 mode=indexing
      tunnel: w3557 -> [w4024] mode=indexing
      tunnel: w3556 -> [w4022]
      tunnel: w3542 -> [w4021]
      n2685 = call "downsample 1D array - double.vi"("Ave N"=w4033, "Array In"=w4034) -> ("Array Out"=w4032:dbl[])  [unwired: 1 out]
      n2686 = Subtract(x=w4032, y=w4024) -> (x-y=w4025:dbl[])
      n2687 = Multiply(x=w4022, y=w4025) -> (x*y=w4023:dbl[])
      n2688 = Multiply(x=w4021, y=w4023) -> (x*y=w4020:dbl[])
      n2689 = Bundle By Name("Y"=w4020, "dt"=w4031, "t0"=w4030) -> (w4029:waveform(dbl))  [unwired: 1 out]
      n2690 = Set Waveform Attribute(5:w4027, 6:w4028, 7:w4029) -> (3:w4026:waveform(dbl))  [unwired: 1 in, 2 out]
    }
    n2691 = Cluster To Array(cluster=w3781) -> (array=w3778:string[])
    n2692 = for "APD" {
      tunnel: w3751 -> [w4381] mode=indexing
      tunnel: w3629 -> [w4389]
      tunnel: [w4385] -> w3636 mode=indexing
      tunnel: "APD Disp. Scale" -> [w4386]
      tunnel: w3601 -> [w4384]
      tunnel: w3778 -> [w4383] mode=indexing
      tunnel: "APD Disp. Downsample" -> [w4379]
      tunnel: [w4382] -> w3777
      workers-P: _ -> [_]
      tunnel: w3602 -> [w4378]
      n2693 = call "integrate 1D array interval - double.vi"("Ave N"=w4379, "Array In"=w4381) -> ("Array Out"=w4380:dbl[])  [unwired: 1 out]
      n2694 = Multiply(x=w4389, y=w4379) -> (x*y=w4382:dbl)
      n2695 = Divide(x=w4380, y=w4386) -> (x/y=w4387:dbl[])
      n2696 = Bundle By Name("t0"=w4378, "Y"=w4387, "dt"=w4382) -> (w4388:waveform(dbl))  [unwired: 1 out]
      n2697 = Set Waveform Attribute(5:w4383, 6:w4384, 7:w4388) -> (3:w4385:waveform(dbl))  [unwired: 1 in, 2 out]
    }
    "APD Display Period (s)" <- w3777
    n2698 = Reciprocal(x=w3777) -> (1/x=→"APD Display Freq. (Hz)":dbl)
    n2699 = local read "Display Period (s)"() -> (w3660:dbl)
    n2700 = Increment(x=w3762) -> (x+1=w3763:dbl)
    n2701 = To Double Precision Float(number=w3672) -> (double precision float=w3671:dbl[])
    n2702 = Index Array(array=w3512, index=0) -> (element=w3516:waveform(dbl))
    n2703 = Index Array(array=w3512, index=1) -> (element=w3511:waveform(dbl))
    n2704 = feedback #11(w3763) -> (w3766:dbl)
    n2705 = Select(t=0, s=w3753, f=w3766) -> (s? t:f=w3759:dbl)
    n2706 = Array Size(array=w3671) -> (size(s)=w3765:i32)
    n2707 = Add(x=w3765, y=w3759) -> (x+y=w3760:dbl)
    n2708 = Unbundle By Name(w3516) -> ("Y"=w3517:dbl[])
    n2709 = feedback #12(w3672) -> (w3749:u32[])
    n2710 = Build Array (concatenate)(w3749, w3672) -> (w3746:u32[])
    n2711 = feedback #13(w3616) -> (w3635:u32[])
    n2712 = Divide(x="Bead Sep. Int. Time (s)", y=w3660) -> (x/y=w3552:dbl)
    n2713 = Build Array (concatenate)(w3635, w3616) -> (w3634:u32[])
    n2714 = Add(x=w3517, y="FB Trap Pos Offset") -> (x+y=w3515:dbl[])
    "T1 x pos data" <- w3515
    n2715 = Greater?(x=w3760, y=w3762) -> (0:w3761:bool)
    n2716 = feedback #14(w3515) -> (w3554:dbl[])
    n2717 = Build Array (concatenate)(w3515, w3554) -> (w3553:dbl[])
    n2718 = Bundle By Name(cluster=w3516, "Y"=w3515) -> (w3514:waveform(dbl))
    n2719 = Select(t=w3759, s=w3761, f=w3760) -> (s? t:f=w3758:dbl)
    n2720 = feedback-in #11(w3758) -> ()
    n2721 = Array Size(array=w3746) -> (size(s)=w3743:i32)
    n2722 = Array Size(array=w3672) -> (size(s)=w3745:i32)
    n2723 = local read "MCL Scanning"() -> (w3756:bool)
    n2724 = local read "APD Integration Time (s)"() -> (w3643:dbl)
    n2725 = Bundle(w3514, w3511) -> (w3510:cluster{waveform(dbl), waveform(dbl)})  [unwired: 1 out]
    n2726 = Build Array (concatenate)(w3636, w3782) -> (w3638:waveform(dbl)[])
    "All Signals" <- w3638
    n2727 = Split 1D Array(array=w3553, index=w3552) -> (first subarray=w3546:dbl[])  [unwired: 1 out]
    n2728 = feedback-in #14(w3546) -> ()
    n2729 = Multiply(x=w3745, y="APD Ave N") -> (x*y=w3744:dbl)
    n2730 = Greater?(x=w3743, y=w3744) -> (0:w3747:bool)
    n2731 = Not(x=w3761) -> (.not. x?=w3755:bool)
    n2732 = Cluster To Array(cluster=w3510) -> (array=w3486:waveform(dbl)[])
    "Trap Positions" <- w3486
    n2733 = To Double Precision Float(number=w3616) -> (double precision float=w3615:dbl[])
    n2734 = call-poly <vilib>:"Mean.vi"("X"=w3546) -> ("mean"=w3545:dbl)  [unwired: 1 out]
    "Mean T1 Position (nm)" <- w3545
    n2735 = Subtract(x=w3546, y=w3545) -> (x-y=w3551:dbl[])
    n2736 = Square(x=w3551) -> (x^2=w3550:dbl[])
    n2737 = And(x=w3755, y=w3756) -> (x .and. y?=w3757:bool)
    n2738 = call-poly <vilib>:"Mean.vi"("X"=w3550) -> ("mean"=w3549:dbl)  [unwired: 1 out]
    n2739 = case shown="True" w3747 {
      tunnel: w3746 -> [w4161 w4168]
      tunnel: [w4161 w4166] -> w3689
      tunnel: w3744 -> [_ w4163]
      tunnel: w3743 -> [_ w4167]
      tunnel: w3634 -> [w4160 w4165]
      tunnel: [w4160 w4162] -> w3631
      frame False {
      }
      frame True {
        n2740 = Subtract(x=w4167, y=w4163) -> (x-y=w4164:dbl)
        n2741 = Array Subset(array=w4168, index=w4164, length=w4163) -> (w4166:u32[])
        n2742 = Array Subset(array=w4165, index=w4164, length=w4163) -> (w4162:u32[])
      }
    }
    n2743 = feedback-in #12(w3689) -> ()
    n2744 = feedback-in #13(w3631) -> ()
    n2745 = Square Root(x=w3549) -> (sqrt(x)=w3548:dbl)
    n2746 = Or(x=w3757, y=w3753) -> (x .or. y?=w3754:bool)
    n2747 = Equal?(x="Tab Control 6", y=T36."High Res Display") -> (x = y?=w3678:bool)
    n2748 = Multiply(x="APD Disp. Scale", y=w3636) -> (x*y=w3645:waveform(dbl)[])
    n2749 = Multiply(x=10.0, y=w3548) -> (x*y=→"Trap 1 Position RMS (A)":dbl)
    n2750 = Multiply(x="APD Disp. Downsample", y=w3643) -> (x*y=w3641:dbl)
    n2751 = Divide(x=w3645, y=w3641) -> (x/y=w3613:waveform(dbl)[])
    n2752 = case "For displaying the high resolution display (no downsampling)" shown="True" w3678 {
      tunnel: w3640 -> [_ w4059]
      frame False {
      }
      frame True {
        n2753 = Index Array(array=w4059, index="High Res. Display") -> (element=w4060:waveform(dbl))
        n2754 = call <vilib>:"Std Deviation and Variance.vi"("X"=w4060) -> ("mean"=w4067:dbl, "standard deviation"=w4072:dbl)  [unwired: 1 in, 1 out]
        "Mean Intensity" <- w4067
        "Sigma" <- w4072
        n2755 = Subtract(x=w4060, y=w4067) -> (x-y=w4066:waveform(dbl))
        n2756 = Select(t=w4066, s="Subtract mean", f=w4060) -> (s? t:f=→"1 Channel":waveform(dbl))
        n2757 = Divide(x=w4072, y=w4067) -> (x/y=→"Sigma/Mean":dbl)
        n2758 = feedback #15(1) -> (w4061:i32)
        n2759 = Greater Or Equal?(x=w4061, y="Slow mean N ave.") -> (x >= y?=w4074:bool)
        n2760 = Increment(x=w4061) -> (x+1=w4076:i32)
        n2761 = Select(t=1, s=w4074, f=w4076) -> (s? t:f=w4063:i32)
        n2762 = feedback-in #15(w4063) -> ()
        n2763 = feedback #16() -> (w4064:waveform(dbl))  [unwired: 1 out]
        n2764 = case shown="Default" w4061 {
          tunnel: [w4079 w4082] -> w4065
          tunnel: w4064 -> [w4081 _]
          tunnel: w4060 -> [w4080 w4082]
          frame Default {
            n2765 = call-poly <vilib>:"Append Waveforms.vi"("waveform B"=w4080, "waveform A"=w4081) -> ("waveform out"=w4079:waveform(dbl))  [unwired: 1 in, 8 out]
          }
          frame 1 {
          }
        }
        n2766 = feedback-in #16(w4065) -> ()
        n2767 = case shown="True" w4074 {
          tunnel: w4065 -> [_ w4078]
          frame False {
          }
          frame True {
            n2768 = call-poly <vilib>:"Mean.vi"("X"=w4078) -> ("mean"=→"Slow mean":dbl)  [unwired: 1 out]
          }
        }
      }
    }
    n2769 = Index Array(array=w3613, index=0) -> (element=w3623:waveform(dbl))
    n2770 = Index Array(array=w3613, index=1) -> (element=w3621:waveform(dbl))
    n2771 = case "For computing FFTs for display" shown="True" "Compute FFT" {
      tunnel: w3640 -> [_ w4775]
      frame False {
      }
      frame True {
        n2772 = Build Array("FFT 1 Choice 1", "FFT 1 Choice 2", "FFT 2 Choice 1", "FFT 2 Choice 2") -> (w4768:u16[])
        n2773 = Array Size(array=w4775) -> (size(s)=w4774:i32)
        n2774 = feedback-in #17(w4768) -> ()
        n2775 = feedback #17(u16[] [100, 100, 100, 100]) -> (w4769:u16[])
        n2776 = feedback-in #18("# Spectra to Ave.") -> ()
        n2777 = feedback #18("# Spectra to Ave.") -> (w4766:dbl)
        n2778 = Not Equal?(x="# Spectra to Ave.", y=w4766) -> (x != y?=w4765:bool)
        n2779 = Not Equal?(x=w4768, y=w4769) -> (x != y?=w4767:bool)
        n2780 = feedback #19(1.0) -> (w4752:dbl)
        n2781 = Compound Arithmetic op=OR("Reset FFT", w4767, w4765) -> (w4750:bool)
        n2782 = Select(t=1.0, s=w4750, f=w4752) -> (s? t:f=w4754:dbl)
        n2783 = Greater?(x=w4754, y="# Spectra to Ave.") -> (0:w4773:bool)
        n2784 = Increment(x=w4754) -> (x+1=w4753:dbl)
        n2785 = feedback-in #19(w4753) -> ()
        n2786 = local read "DMA Update Period (s)"() -> (w4748:dbl)
        n2787 = Multiply(x="# Spectra to Ave.", y=w4748) -> (x*y=→"Ave. Time (s)":dbl)
        n2788 = Build Array(cluster{"f0":dbl, "df":dbl, "magnitude":dbl[]} {"f0"=0.0, "df"=0.0, "magnitude"=[]} ("PSD")) -> (w4757:cluster{"f0":dbl, "df":dbl, "magnitude":dbl[]}[])
        n2789 = Build Array(w4757, w4757, w4757, w4757) -> (w4759:T47)
        n2790 = feedback #20(w4759) -> (w4764:T47)
        n2791 = for {
          N: 4 -> [_]
          tunnel: w4768 -> [w4797] mode=indexing
          tunnel: w4775 -> [w4798]
          tunnel: w4774 -> [w4800]
          tunnel: w4750 -> [w4793]
          tunnel: w4773 -> [w4792]
          tunnel: "# Spectra to Ave." -> [w4791]
          tunnel: [w4790] -> w4763 mode=indexing
          tunnel: w4764 -> [w4795] mode=indexing
          tunnel: [w4794] -> w4751 mode=indexing
          tunnel: w4754 -> [w4789]
          n2792 = Less?(x=w4797, y=w4800) -> (x < y?=w4799:bool)
          n2793 = Index Array(array=w4798, index=w4797) -> (element=w4796:waveform(dbl))
          n2794 = case shown="True" w4799 {
            tunnel: w4796 -> [_ w4817]
            tunnel: w4795 -> [w4802 w4815]
            tunnel: [w4802 w4803] -> w4794
            tunnel: w4793 -> [_ w4814]
            tunnel: w4792 -> [_ w4807]
            tunnel: w4791 -> [_ w4806]
            tunnel: [cluster{"f0":dbl, "df":dbl, "magnitude":dbl[]} {"f0"=0.0, "df"=0.0, "magnitude"=[]} ("PSD") w4808] -> w4790
            tunnel: w4789 -> [_ w4805]
            frame False {
            }
            frame True {
              n2795 = call <vilib>:"Std Deviation and Variance.vi"("X"=w4817) -> ("mean"=w4818:dbl)  [unwired: 1 in, 2 out]
              n2796 = Subtract(x=w4817, y=w4818) -> (x-y=w4816:waveform(dbl))
              n2797 = xnode "Spectral Measurements"("Signals"=w4816) -> ("PSD"=w4810:cluster{"f0":dbl, "df":dbl, "magnitude":dbl[]})  [unwired: 1 in, 1 out]
              n2798 = case shown="False" w4814 {
                tunnel: w4815 -> [w4827 _]
                tunnel: [w4823 w4832] -> w4803
                tunnel: w4810 -> [w4826 w4833]
                tunnel: w4807 -> [w4825 _]
                frame False {
                  n2799 = Build Array (concatenate)(w4827, w4826) -> (w4824:cluster{"f0":dbl, "df":dbl, "magnitude":dbl[]}[])
                  n2800 = case shown="True" w4825 {
                    tunnel: w4824 -> [w4828 w4831]
                    tunnel: [w4828 w4829] -> w4823
                    frame False {
                    }
                    frame True {
                      n2801 = Delete From Array(array=w4831, index=0) -> (array with subset deleted=w4829:cluster{"f0":dbl, "df":dbl, "magnitude":dbl[]}[])  [unwired: 1 in, 1 out]
                    }
                  }
                }
                frame True {
                  n2802 = Build Array(w4833) -> (w4832:cluster{"f0":dbl, "df":dbl, "magnitude":dbl[]}[])
                }
              }
              n2803 = for {
                tunnel: w4803 -> [w4822] mode=indexing
                tunnel: [w4821] -> w4813 mode=indexing
                workers-P: _ -> [_]
                n2804 = Unbundle By Name(w4822) -> ("magnitude"=w4821:dbl[])
              }
              n2805 = Transpose 2D Array(2D array=w4813) -> (transposed array=w4812:dbl[][])
              n2806 = for {
                tunnel: w4812 -> [w4820] mode=indexing
                tunnel: [w4819] -> w4811 mode=indexing
                workers-P: _ -> [_]
                n2807 = Add Array Elements(numeric array=w4820) -> (sum=w4819:dbl)
              }
              n2808 = Select(t=w4806, s=w4807, f=w4805) -> (s? t:f=w4804:dbl)
              n2809 = Divide(x=w4811, y=w4804) -> (x/y=w4809:dbl[])
              n2810 = Bundle By Name(cluster=w4810, "magnitude"=w4809) -> (w4808:cluster{"f0":dbl, "df":dbl, "magnitude":dbl[]})
            }
          }
        }
        n2811 = case shown="True" w4750 {
          tunnel: w4751 -> [w4782 w4788]
          tunnel: [w4782 w4783] -> w4749
          frame False {
          }
          frame True {
            n2812 = Array Subset(array=w4788, index (row)=0 ("index"), length (row)=4 ("length"), index (col)=0 ("index"), length (col)=1 ("length")) -> (w4783:T47)
          }
        }
        n2813 = feedback-in #20(w4749) -> ()
        n2814 = Split 1D Array(array=w4763, index=2) -> (first subarray=→"FFT 1":cluster{"f0":dbl, "df":dbl, "magnitude":dbl[]}[], second subarray=→"FFT 2":cluster{"f0":dbl, "df":dbl, "magnitude":dbl[]}[])
      }
    }
    n2815 = case "For plotting results of scanning MCL" shown="True" w3754 {
      tunnel: w3753 -> [_ w4201]
      tunnel: w3671 -> [_ w4297]
      tunnel: w3762 -> [_ _]
      tunnel: w3640 -> [_ w4271]
      tunnel: w3615 -> [_ w4202]
      tunnel: w3614 -> [_ w4175]
      frame False {
      }
      frame True {
        w4182 = u32 0 items=["Horizontal", "Vertical", "Central", "1st Diagonal", "2nd Diagonal"] ("Type of Symmetry")
        w4210 = u32 0 items=["Horizontal", "Vertical", "Central", "1st Diagonal", "2nd Diagonal"] ("Type of Symmetry")
        w4213 = u32 0 items=["Horizontal", "Vertical", "Central", "1st Diagonal", "2nd Diagonal"] ("Type of Symmetry")
        w4242 = u32 0 items=["Horizontal", "Vertical", "Central", "1st Diagonal", "2nd Diagonal"] ("Type of Symmetry")
        n2816 = Index Array(array=w4271, index=10) -> (element=w4277:waveform(dbl))
        n2817 = Index Array(array=w4271, index=11) -> (element=w4274:waveform(dbl))
        n2818 = local read "Cycles/step (MCL)"() -> (w4227:u64)
        n2819 = Index Array(array=w4271, index="Channel") -> (element=w4273:waveform(dbl))
        n2820 = Unbundle(w4175) -> ("New Image"=w4174:T2, "New Image"=w4173:T2, "New Image"=w4172:T2, "New Image"=w4171:T2)
        n2821 = Unbundle By Name(w4277) -> ("Y"=w4229:dbl[])
        n2822 = Unbundle By Name(w4274) -> ("Y"=w4231:dbl[])
        n2823 = Unbundle By Name(w4273) -> ("Y"=w4236:dbl[])
        n2824 = call "downsample 1D array - double.vi"("Ave N"=w4227, "Array In"=w4229) -> ("Array Out"=w4228:dbl[])  [unwired: 1 out]
        n2825 = call "downsample 1D array - double.vi"("Ave N"=w4227, "Array In"=w4231) -> ("Array Out"=w4230:dbl[])  [unwired: 1 out]
        n2826 = call "downsample 1D array - double.vi"("Ave N"=w4227, "Array In"=w4236) -> ("Array Out"=w4235:dbl[])  [unwired: 1 out]
        n2827 = feedback #21(w4297) -> (w4298:dbl[])
        n2828 = Build Array (concatenate)(w4298, w4297) -> (w4279:dbl[])
        n2829 = feedback #22(w4202) -> (w4204:dbl[])
        n2830 = Build Array (concatenate)(w4204, w4202) -> (w4203:dbl[])
        n2831 = local read "Scan steps (MCL)"() -> (w4184:u64)
        n2832 = Select(t=w4297, s=w4201, f=w4279) -> (s? t:f=w4283:dbl[])
        n2833 = feedback-in #21(w4283) -> ()
        n2834 = Select(t=w4202, s=w4201, f=w4203) -> (s? t:f=w4185:dbl[])
        n2835 = feedback-in #22(w4185) -> ()
        n2836 = local read "Scan lines (y)"() -> (w4170:u64)
        n2837 = local read "N APD Samp/step"() -> (w4186:dbl)
        n2838 = feedback #23(w4228) -> (w4285:dbl[])
        n2839 = Build Array (concatenate)(w4285, w4228) -> (w4276:dbl[])
        n2840 = feedback #24(w4235) -> (w4295:dbl[])
        n2841 = Build Array (concatenate)(w4295, w4235) -> (w4294:dbl[])
        n2842 = feedback #25(w4230) -> (w4287:dbl[])
        n2843 = Build Array (concatenate)(w4287, w4230) -> (w4288:dbl[])
        n2844 = Select(t=w4228, s=w4201, f=w4276) -> (s? t:f=w4232:dbl[])
        n2845 = feedback-in #23(w4232) -> ()
        n2846 = Select(t=w4235, s=w4201, f=w4294) -> (s? t:f=w4234:dbl[])
        n2847 = feedback-in #24(w4234) -> ()
        n2848 = Select(t=w4230, s=w4201, f=w4288) -> (s? t:f=w4233:dbl[])
        n2849 = feedback-in #25(w4233) -> ()
